vi "Logs.vi"(8 "error in":errorcluster, 10 "Action":enum16{"GetList", "AddRecord", "ClearList"}(ring), 11 "Cluster":cluster{"Log":string, "Time Stamp":timestamp}) -> (0 "error out":errorcluster, 3 "Logs":string)   [LabVIEW 2022 SP3]
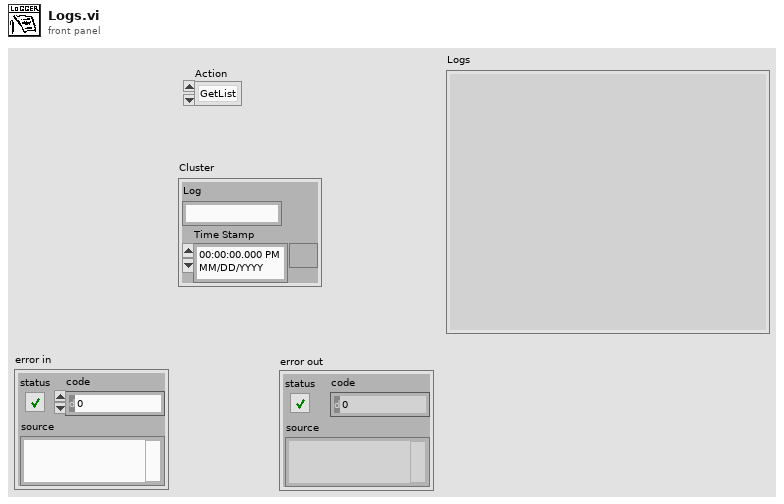
[diagram p1: front panel]
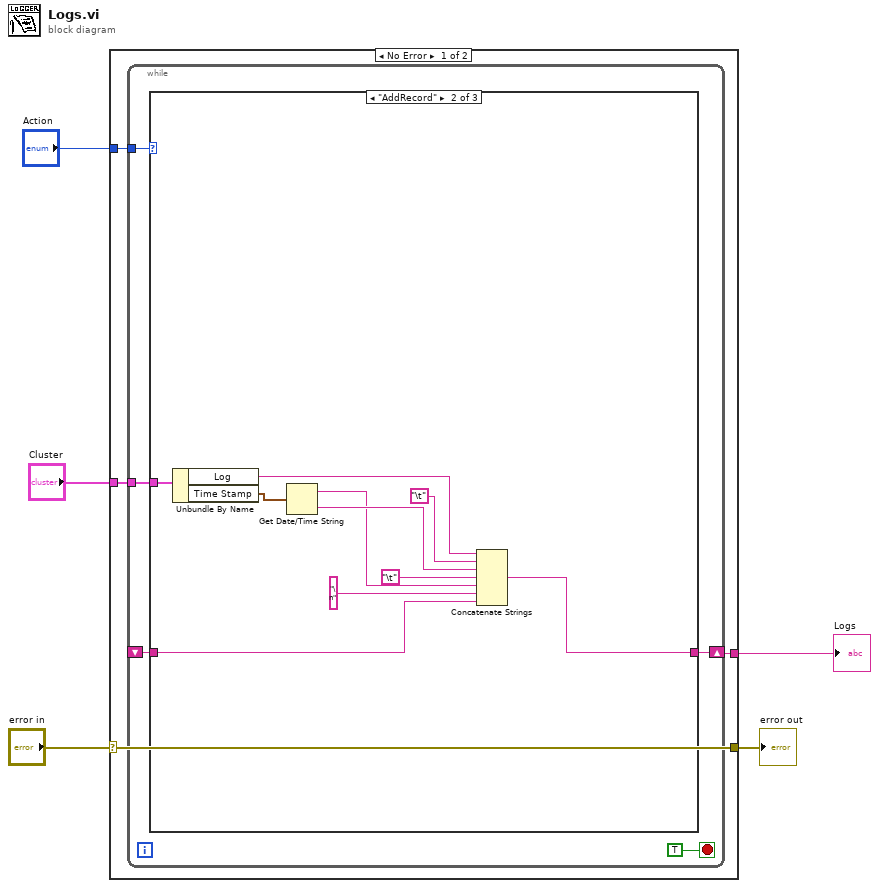
[diagram p0: block diagram]
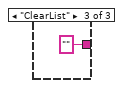
[diagram p3: hidden frame]
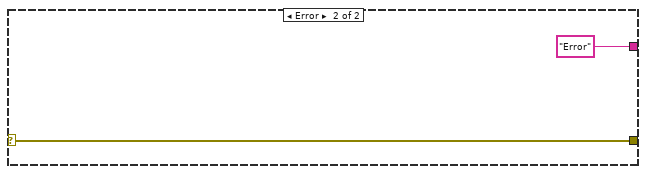
[diagram p4: hidden frame]
diagram:
  n1 = case shown="No Error" "error in" {
    selector: "error in" -> [w9 w28]
    tunnel: [w9 w28] -> w4
    tunnel: "Action" -> [w8 _]
    tunnel: [w7 "Error"] -> w2
    tunnel: "Cluster" -> [w6 _]
    frame No Error {
      n2 = while {
        tunnel: w8 -> [w13]
        shift-right: [w10] -> w7
        shift-left: _ -> [w11]
        tunnel: w6 -> [w12]
        stop <- TRUE stop-if-true
        n3 = case shown="\"AddRecord\"" w13 {
          tunnel: w12 -> [_ w25 _]
          tunnel: w11 -> [w15 w16 _]
          tunnel: [w15 w18 ""] -> w10
          frame "GetList", Default {
          }
          frame "AddRecord" {
            n4 = Unbundle By Name(w25) -> ("Log"=w23:string, "Time Stamp"=w24:timestamp)
            n5 = Get Date/Time String(seconds (now)=w24) -> (date string=w19:string, time string=w21:string)  [unwired: 2 in]
            n6 = Concatenate Strings(w23, "\t" ("string"), w21, "\t" ("string"), w19, "\n" ("string"), w16) -> (w18:string)
          }
          frame "ClearList" {
          }
        }
      }
    }
    frame Error {
    }
  }
  "error out" <- w4
  "Logs" <- w2
